vi "niFpga wdp fft streaming bf core.vi"(4 "index=0?":bool, 6 "enable":bool, 8 "switch":bool[](array[boolean])=[FALSE, FALSE, FALSE, FALSE, FALSE, FALSE, FALSE, FALSE, FALSE, FALSE, FALSE, FALSE, FALSE, FALSE, FALSE], 9 "twiddle factors":T1(array[cluster])=[{"tf re"=0.0, "tf im"=0.0}, {"tf re"=0.0, "tf im"=0.0}], 10 "data in 1":T3, 11 "data in 0":T3) -> (2 "data out 1":T2, 3 "data out 0":T2)   [LabVIEW 2017]
types:
  T1 = cluster{"tf re":fxp<+/-,16,16>, "tf im":fxp<+/-,16,16>}[]
  T2 = cluster{"data re":fxp<+/-,23,16>, "data re":fxp<+/-,23,16>}
  T3 = cluster{"data re":fxp<+/-,16,16>, "data im":fxp<+/-,16,16>}
  T4 = cluster{"tf re":fxp<+/-,16,16>, "tf im":fxp<+/-,16,16>}
  T5 = cluster{"data re":fxp<+/-,8,1>, "data re":fxp<+/-,8,1>}
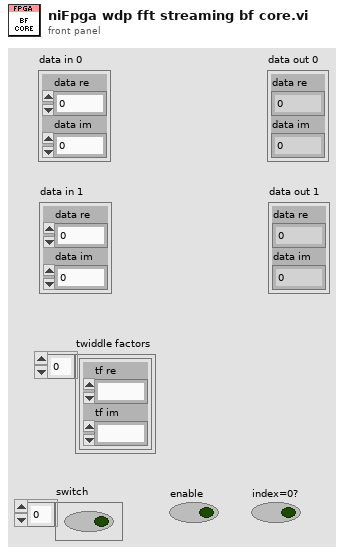
[diagram p1: front panel]
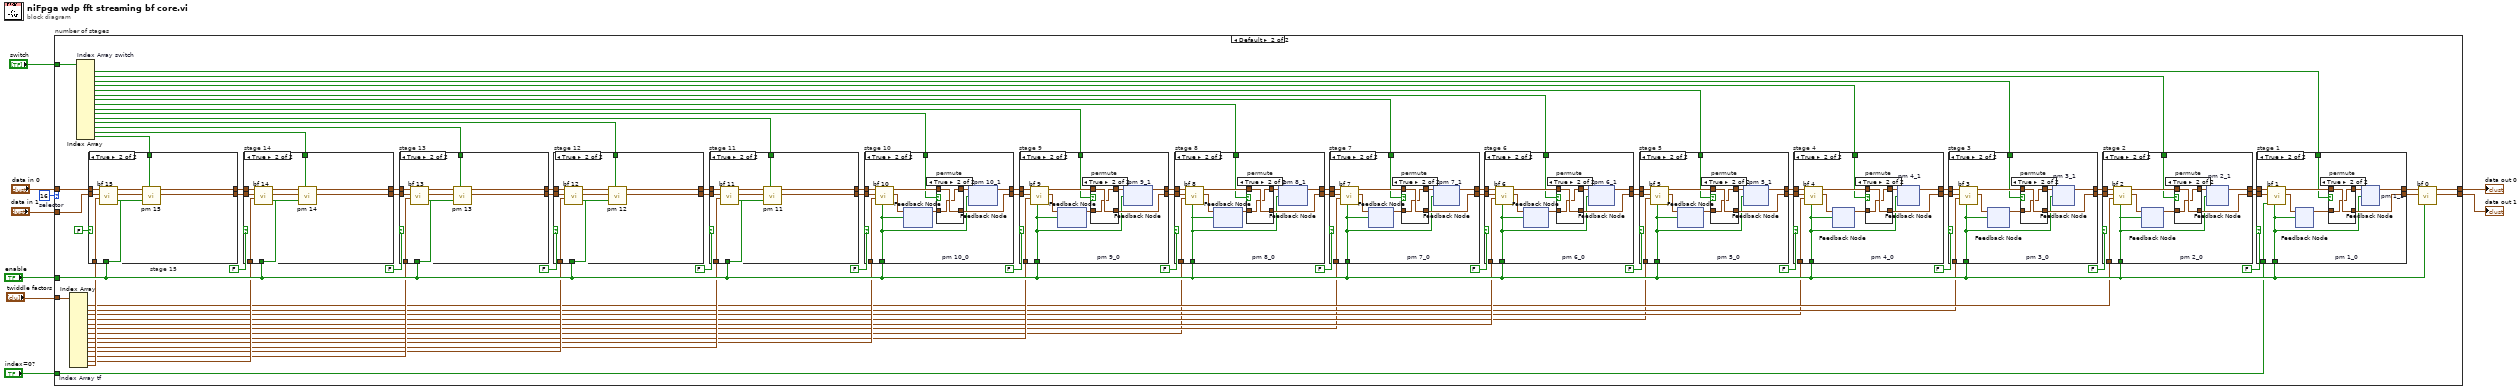
[diagram p0: block diagram]
diagram:
  w6 = u8 16  # selector
  n1 = case "number of stages" shown="Default" w6 {
    tunnel: "data in 0" -> [w11 w90]
    tunnel: "data in 1" -> [w10 w89]
    tunnel: "enable" -> [_ w56]
    tunnel: "twiddle factors" -> [_ w93]
    tunnel: "switch" -> [_ w92]
    tunnel: [w11 w58] -> w2
    tunnel: [w10 w57] -> w1
    tunnel: "index=0?" -> [_ w41]
    frame 0 {
    }
    frame Default {
      n2 = Index Array "Index Array tf"(array=w93) -> (element #1=w47:T4, element #2=w46:T4, element #3=w45:T4, element #4=w44:T4, element #5=w48:T4, element #6=w43:T4, element #7=w42:T4, element #8=w49:T4, element #9=w50:T4, element #10=w51:T4, element #11=w52:T4, element #12=w53:T4, element #13=w54:T4, element #14=w55:T4)  [unwired: 14 in]
      n3 = Index Array "Index Array switch"(array=w92) -> (element #1=w27:bool, element #2=w28:bool, element #3=w29:bool, element #4=w30:bool, element #5=w31:bool, element #6=w32:bool, element #7=w33:bool, element #8=w34:bool, element #9=w35:bool, element #10=w36:bool, element #11=w37:bool, element #12=w38:bool, element #13=w39:bool, element #14=w40:bool, element #15=w91:bool)  [unwired: 15 in]
      n4 = case "stage 15" shown="True" FALSE {
        tunnel: w90 -> [w309 w318]
        tunnel: w89 -> [w308 w317]
        tunnel: w55 -> [_ w316]
        tunnel: [w309 w312] -> w88
        tunnel: [w308 w311] -> w87
        tunnel: w91 -> [_ w313]
        tunnel: w56 -> [_ w310]
        frame False {
        }
        frame True {
          n5 = call "bf 15"("enable"=w310, "twiddle factor"=w316, "data in 1"=w317, "data in 0"=w318) -> ("data out 1"=w314:T5, "data out 0"=w315:T5)  [unwired: 6 in]
          n6 = call "pm 15"("enable"=w310, "switch"=w313, "data in 1"=w314, "data in 0"=w315) -> ("data out 1"=w311:T5, "data out 0"=w312:cluster{fxp<+/-,8,1>, fxp<+/-,8,1>})  [unwired: 6 in]
        }
      }
      n7 = case "stage 14" shown="True" FALSE {
        tunnel: w88 -> [w298 w307]
        tunnel: w87 -> [w297 w306]
        tunnel: w54 -> [_ w305]
        tunnel: [w298 w301] -> w86
        tunnel: [w297 w300] -> w85
        tunnel: w40 -> [_ w302]
        tunnel: w56 -> [_ w299]
        frame False {
        }
        frame True {
          n8 = call "bf 14"("enable"=w299, "twiddle factor"=w305, "data in 1"=w306, "data in 0"=w307) -> ("data out 1"=w303:T5, "data out 0"=w304:T5)  [unwired: 6 in]
          n9 = call "pm 14"("enable"=w299, "switch"=w302, "data in 1"=w303, "data in 0"=w304) -> ("data out 1"=w300:T5, "data out 0"=w301:cluster{fxp<+/-,8,1>, fxp<+/-,8,1>})  [unwired: 6 in]
        }
      }
      n10 = case "stage 13" shown="True" FALSE {
        tunnel: w86 -> [w287 w296]
        tunnel: w85 -> [w286 w295]
        tunnel: w53 -> [_ w294]
        tunnel: [w287 w290] -> w84
        tunnel: [w286 w289] -> w83
        tunnel: w39 -> [_ w291]
        tunnel: w56 -> [_ w288]
        frame False {
        }
        frame True {
          n11 = call "bf 13"("enable"=w288, "twiddle factor"=w294, "data in 1"=w295, "data in 0"=w296) -> ("data out 1"=w292:T5, "data out 0"=w293:T5)  [unwired: 6 in]
          n12 = call "pm 13"("enable"=w288, "switch"=w291, "data in 1"=w292, "data in 0"=w293) -> ("data out 1"=w289:T5, "data out 0"=w290:cluster{fxp<+/-,8,1>, fxp<+/-,8,1>})  [unwired: 6 in]
        }
      }
      n13 = case "stage 12" shown="True" FALSE {
        tunnel: w84 -> [w276 w285]
        tunnel: w83 -> [w275 w284]
        tunnel: w52 -> [_ w283]
        tunnel: [w276 w279] -> w82
        tunnel: [w275 w278] -> w81
        tunnel: w38 -> [_ w280]
        tunnel: w56 -> [_ w277]
        frame False {
        }
        frame True {
          n14 = call "bf 12"("enable"=w277, "twiddle factor"=w283, "data in 1"=w284, "data in 0"=w285) -> ("data out 1"=w281:T5, "data out 0"=w282:T5)  [unwired: 6 in]
          n15 = call "pm 12"("enable"=w277, "switch"=w280, "data in 1"=w281, "data in 0"=w282) -> ("data out 1"=w278:T5, "data out 0"=w279:cluster{fxp<+/-,8,1>, fxp<+/-,8,1>})  [unwired: 6 in]
        }
      }
      n16 = case "stage 11" shown="True" FALSE {
        tunnel: w82 -> [w265 w274]
        tunnel: w81 -> [w264 w273]
        tunnel: w51 -> [_ w272]
        tunnel: [w265 w268] -> w80
        tunnel: [w264 w267] -> w79
        tunnel: w37 -> [_ w269]
        tunnel: w56 -> [_ w266]
        frame False {
        }
        frame True {
          n17 = call "bf 11"("enable"=w266, "twiddle factor"=w272, "data in 1"=w273, "data in 0"=w274) -> ("data out 1"=w270:T5, "data out 0"=w271:T5)  [unwired: 6 in]
          n18 = call "pm 11"("enable"=w266, "switch"=w269, "data in 1"=w270, "data in 0"=w271) -> ("data out 1"=w267:T5, "data out 0"=w268:cluster{fxp<+/-,8,1>, fxp<+/-,8,1>})  [unwired: 6 in]
        }
      }
      n19 = case "stage 10" shown="True" FALSE {
        tunnel: w80 -> [w248 w259]
        tunnel: w79 -> [w247 w258]
        tunnel: w50 -> [_ w257]
        tunnel: [w248 w253] -> w78
        tunnel: [w247 w252] -> w77
        tunnel: w36 -> [_ w254]
        tunnel: w56 -> [_ w251]
        frame False {
        }
        frame True {
          n20 = call "bf 10"("enable"=w251, "twiddle factor"=w257, "data in 1"=w258, "data in 0"=w259) -> ("data out 1"=w255:T5, "data out 0"=w256:T5)  [unwired: 6 in]
          n21 = feedback #1 "pm 10_0"() -> (w250:T5)  [unwired: 1 in]
          n22 = feedback-in #1(w255, w251) -> ()
          n23 = case "permute" shown="True" w254 {
            tunnel: w256 -> [w261 w263]
            tunnel: [w260 w263] -> w252
            tunnel: [w261 w262] -> w249
            tunnel: w250 -> [w260 w262]
            frame False {
            }
            frame True {
            }
          }
          n24 = feedback #2 "pm 10_1"() -> (w253:T5)  [unwired: 1 in]
          n25 = feedback-in #2(w249, w251) -> ()
        }
      }
      n26 = case "stage 9" shown="True" FALSE {
        tunnel: w78 -> [w231 w242]
        tunnel: w77 -> [w230 w241]
        tunnel: w49 -> [_ w240]
        tunnel: [w231 w236] -> w76
        tunnel: [w230 w235] -> w75
        tunnel: w35 -> [_ w237]
        tunnel: w56 -> [_ w234]
        frame False {
        }
        frame True {
          n27 = call "bf 9"("enable"=w234, "twiddle factor"=w240, "data in 1"=w241, "data in 0"=w242) -> ("data out 1"=w238:T5, "data out 0"=w239:T5)  [unwired: 6 in]
          n28 = feedback #3 "pm 9_0"() -> (w233:T5)  [unwired: 1 in]
          n29 = feedback-in #3(w238, w234) -> ()
          n30 = case "permute" shown="True" w237 {
            tunnel: w239 -> [w244 w246]
            tunnel: [w243 w246] -> w235
            tunnel: [w244 w245] -> w232
            tunnel: w233 -> [w243 w245]
            frame False {
            }
            frame True {
            }
          }
          n31 = feedback #4 "pm 9_1"() -> (w236:T5)  [unwired: 1 in]
          n32 = feedback-in #4(w232, w234) -> ()
        }
      }
      n33 = case "stage 8" shown="True" FALSE {
        tunnel: w76 -> [w214 w225]
        tunnel: w75 -> [w213 w224]
        tunnel: w42 -> [_ w223]
        tunnel: [w214 w219] -> w74
        tunnel: [w213 w218] -> w73
        tunnel: w34 -> [_ w220]
        tunnel: w56 -> [_ w217]
        frame False {
        }
        frame True {
          n34 = call "bf 8"("enable"=w217, "twiddle factor"=w223, "data in 1"=w224, "data in 0"=w225) -> ("data out 1"=w221:T5, "data out 0"=w222:T5)  [unwired: 6 in]
          n35 = feedback #5 "pm 8_0"() -> (w216:T5)  [unwired: 1 in]
          n36 = feedback-in #5(w221, w217) -> ()
          n37 = case "permute" shown="True" w220 {
            tunnel: w222 -> [w227 w229]
            tunnel: [w226 w229] -> w218
            tunnel: [w227 w228] -> w215
            tunnel: w216 -> [w226 w228]
            frame False {
            }
            frame True {
            }
          }
          n38 = feedback #6 "pm 8_1"() -> (w219:T5)  [unwired: 1 in]
          n39 = feedback-in #6(w215, w217) -> ()
        }
      }
      n40 = case "stage 7" shown="True" FALSE {
        tunnel: w74 -> [w197 w208]
        tunnel: w73 -> [w196 w207]
        tunnel: w43 -> [_ w206]
        tunnel: [w197 w202] -> w72
        tunnel: [w196 w201] -> w71
        tunnel: w33 -> [_ w203]
        tunnel: w56 -> [_ w200]
        frame False {
        }
        frame True {
          n41 = call "bf 7"("enable"=w200, "twiddle factor"=w206, "data in 1"=w207, "data in 0"=w208) -> ("data out 1"=w204:T5, "data out 0"=w205:T5)  [unwired: 6 in]
          n42 = feedback #7 "pm 7_0"() -> (w199:T5)  [unwired: 1 in]
          n43 = feedback-in #7(w204, w200) -> ()
          n44 = case "permute" shown="True" w203 {
            tunnel: w205 -> [w210 w212]
            tunnel: [w209 w212] -> w201
            tunnel: [w210 w211] -> w198
            tunnel: w199 -> [w209 w211]
            frame False {
            }
            frame True {
            }
          }
          n45 = feedback #8 "pm 7_1"() -> (w202:T5)  [unwired: 1 in]
          n46 = feedback-in #8(w198, w200) -> ()
        }
      }
      n47 = case "stage 6" shown="True" FALSE {
        tunnel: w72 -> [w180 w191]
        tunnel: w71 -> [w179 w190]
        tunnel: w48 -> [_ w189]
        tunnel: [w180 w185] -> w70
        tunnel: [w179 w184] -> w69
        tunnel: w32 -> [_ w186]
        tunnel: w56 -> [_ w183]
        frame False {
        }
        frame True {
          n48 = call "bf 6"("enable"=w183, "twiddle factor"=w189, "data in 1"=w190, "data in 0"=w191) -> ("data out 1"=w187:T5, "data out 0"=w188:T5)  [unwired: 6 in]
          n49 = feedback #9 "pm 6_0"() -> (w182:T5)  [unwired: 1 in]
          n50 = feedback-in #9(w187, w183) -> ()
          n51 = case "permute" shown="True" w186 {
            tunnel: w188 -> [w193 w195]
            tunnel: [w192 w195] -> w184
            tunnel: [w193 w194] -> w181
            tunnel: w182 -> [w192 w194]
            frame False {
            }
            frame True {
            }
          }
          n52 = feedback #10 "pm 6_1"() -> (w185:T5)  [unwired: 1 in]
          n53 = feedback-in #10(w181, w183) -> ()
        }
      }
      n54 = case "stage 5" shown="True" FALSE {
        tunnel: w70 -> [w163 w174]
        tunnel: w69 -> [w162 w173]
        tunnel: w44 -> [_ w172]
        tunnel: [w163 w168] -> w68
        tunnel: [w162 w167] -> w67
        tunnel: w31 -> [_ w169]
        tunnel: w56 -> [_ w166]
        frame False {
        }
        frame True {
          n55 = call "bf 5"("enable"=w166, "twiddle factor"=w172, "data in 1"=w173, "data in 0"=w174) -> ("data out 1"=w170:T5, "data out 0"=w171:T5)  [unwired: 6 in]
          n56 = feedback #11 "pm 5_0"() -> (w165:T5)  [unwired: 1 in]
          n57 = feedback-in #11(w170, w166) -> ()
          n58 = case "permute" shown="True" w169 {
            tunnel: w171 -> [w176 w178]
            tunnel: [w175 w178] -> w167
            tunnel: [w176 w177] -> w164
            tunnel: w165 -> [w175 w177]
            frame False {
            }
            frame True {
            }
          }
          n59 = feedback #12 "pm 5_1"() -> (w168:T5)  [unwired: 1 in]
          n60 = feedback-in #12(w164, w166) -> ()
        }
      }
      n61 = case "stage 4" shown="True" FALSE {
        tunnel: w68 -> [w146 w157]
        tunnel: w67 -> [w145 w156]
        tunnel: w45 -> [_ w155]
        tunnel: [w146 w151] -> w66
        tunnel: [w145 w150] -> w65
        tunnel: w30 -> [_ w152]
        tunnel: w56 -> [_ w149]
        frame False {
        }
        frame True {
          n62 = call "bf 4"("enable"=w149, "twiddle factor"=w155, "data in 1"=w156, "data in 0"=w157) -> ("data out 1"=w153:T5, "data out 0"=w154:T5)  [unwired: 6 in]
          n63 = feedback #13 "pm 4_0"() -> (w148:T5)  [unwired: 1 in]
          n64 = feedback-in #13(w153, w149) -> ()
          n65 = case "permute" shown="True" w152 {
            tunnel: w154 -> [w159 w161]
            tunnel: [w158 w161] -> w150
            tunnel: [w159 w160] -> w147
            tunnel: w148 -> [w158 w160]
            frame False {
            }
            frame True {
            }
          }
          n66 = feedback #14 "pm 4_1"() -> (w151:T5)  [unwired: 1 in]
          n67 = feedback-in #14(w147, w149) -> ()
        }
      }
      n68 = case "stage 3" shown="True" FALSE {
        tunnel: w66 -> [w129 w140]
        tunnel: w65 -> [w128 w139]
        tunnel: w46 -> [_ w138]
        tunnel: [w129 w134] -> w64
        tunnel: [w128 w133] -> w63
        tunnel: w29 -> [_ w135]
        tunnel: w56 -> [_ w132]
        frame False {
        }
        frame True {
          n69 = call "bf 3"("enable"=w132, "twiddle factor"=w138, "data in 1"=w139, "data in 0"=w140) -> ("data out 1"=w136:T5, "data out 0"=w137:T5)  [unwired: 6 in]
          n70 = feedback #15 "pm 3_0"() -> (w131:T5)  [unwired: 1 in]
          n71 = feedback-in #15(w136, w132) -> ()
          n72 = case "permute" shown="True" w135 {
            tunnel: w137 -> [w142 w144]
            tunnel: [w141 w144] -> w133
            tunnel: [w142 w143] -> w130
            tunnel: w131 -> [w141 w143]
            frame False {
            }
            frame True {
            }
          }
          n73 = feedback #16 "pm 3_1"() -> (w134:T5)  [unwired: 1 in]
          n74 = feedback-in #16(w130, w132) -> ()
        }
      }
      n75 = case "stage 2" shown="True" FALSE {
        tunnel: w64 -> [w112 w123]
        tunnel: w63 -> [w111 w122]
        tunnel: w47 -> [_ w121]
        tunnel: [w112 w117] -> w62
        tunnel: [w111 w116] -> w61
        tunnel: w28 -> [_ w118]
        tunnel: w56 -> [_ w115]
        frame False {
        }
        frame True {
          n76 = call "bf 2"("enable"=w115, "twiddle factor"=w121, "data in 1"=w122, "data in 0"=w123) -> ("data out 1"=w119:T5, "data out 0"=w120:T5)  [unwired: 6 in]
          n77 = feedback #17 "pm 2_0"() -> (w114:T5)  [unwired: 1 in]
          n78 = feedback-in #17(w119, w115) -> ()
          n79 = case "permute" shown="True" w118 {
            tunnel: w120 -> [w125 w127]
            tunnel: [w124 w127] -> w116
            tunnel: [w125 w126] -> w113
            tunnel: w114 -> [w124 w126]
            frame False {
            }
            frame True {
            }
          }
          n80 = feedback #18 "pm 2_1"() -> (w117:T5)  [unwired: 1 in]
          n81 = feedback-in #18(w113, w115) -> ()
        }
      }
      n82 = case "stage 1" shown="True" FALSE {
        tunnel: w62 -> [w95 w106]
        tunnel: w61 -> [w94 w105]
        tunnel: [w95 w101] -> w60
        tunnel: [w94 w100] -> w59
        tunnel: w27 -> [_ w102]
        tunnel: w56 -> [_ w99]
        tunnel: w41 -> [_ w98]
        frame False {
        }
        frame True {
          n83 = call "bf 1"("enable"=w99, "index=0?"=w98, "data in 1"=w105, "data in 0"=w106) -> ("data out 1"=w103:T5, "data out 0"=w104:T5)  [unwired: 6 in]
          n84 = feedback #19 "pm 1_0"() -> (w97:T5)  [unwired: 1 in]
          n85 = feedback-in #19(w103, w99) -> ()
          n86 = case "permute" shown="True" w102 {
            tunnel: w104 -> [w108 w110]
            tunnel: [w107 w110] -> w100
            tunnel: [w108 w109] -> w96
            tunnel: w97 -> [w107 w109]
            frame False {
            }
            frame True {
            }
          }
          n87 = feedback #20 "pm 1_1"() -> (w101:T5)  [unwired: 1 in]
          n88 = feedback-in #20(w96, w99) -> ()
        }
      }
      n89 = call "bf 0"("enable"=w56, "data in 1"=w59, "data in 0"=w60) -> ("data out 1"=w57:T5, "data out 0"=w58:T5)  [unwired: 7 in]
    }
  }
  "data out 0" <- w2
  "data out 1" <- w1
